vi "read_attributes.vi"(8 "error in (no error)":errorcluster, 11 "VotingClassifier in":refnum<class "VotingClassifier.lvclass">) -> (0 "error out":errorcluster, 2 "attributes":T1, 3 "VotingClassifier out":refnum<class "VotingClassifier.lvclass">)   [LabVIEW 2020, in "VotingClassifier.lvclass"]
uses:
  VotingClassifier.lvclass
  Controls/voting_classifier_attributes.ctl
  VotingClassifier.lvclass/VotingClassifier.ctl
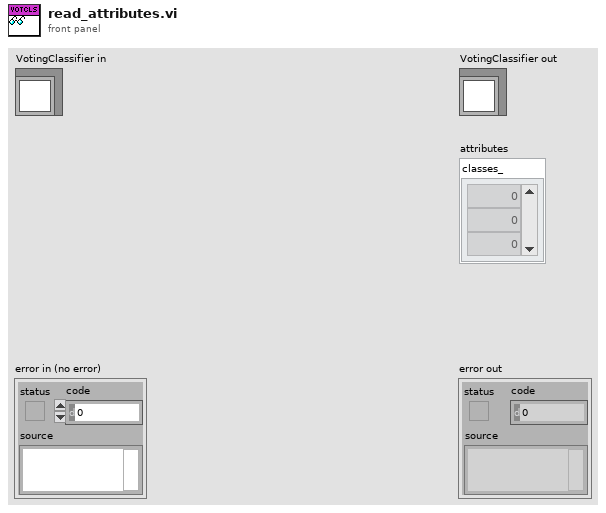
[diagram p1: front panel]
types:
  T1 = typedef "voting_classifier_attributes.ctl" = cluster{"classes_":dbl[]}
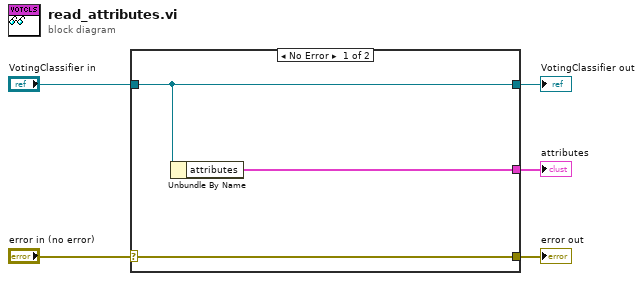
[diagram p0: block diagram]
diagram:
  n1 = case shown="No Error" "error in (no error)" {
    selector: "error in (no error)" -> [w8 w9]
    tunnel: [w8 w9] -> w4
    tunnel: [w7 w10] -> w2
    tunnel: "VotingClassifier in" -> [w7 w10]
    tunnel: [w6 _] -> w1
    frame No Error {
      n2 = Unbundle By Name(w7) -> ("attributes"=w6:T1)
    }
    frame Error {
    }
  }
  "error out" <- w4
  "VotingClassifier out" <- w2
  "attributes" <- w1
